vi "Read image data.vi"() -> ()   [LabVIEW 2020, in "sqlite3.lvlib"]
uses:
  sqlite3.lvlib
  sqlite/VIs/open v2.vi
  sqlite/VIs/prepare v2.vi
  sqlite/VIs/step.vi
  sqlite/VIs/column count.vi
  compound/Column.vi
  compound/Resolve Result Type.vi
  sqlite/VIs/finalize.vi
  sqlite/VIs/close v2.vi
  sqlite/subvi/Error Converter (ErrCode or Status).vi
  sqlite/VIs/column text.vi
  sqlite/VIs/column bytes.vi
  sqlite/VIs/column blob.vi
  utilities/MoveBlock.vi
  sqlite/VIs/column type.vi
  sqlite/VIs/errstr.vi
panel:
  in  "id value":string
  in  "id col":string="image"
  in  "blob column name":string="image"
  in  "table name":string="blob"
  in  "error in (no error)":errorcluster
  out "error out":errorcluster={"status"=TRUE, "code"=43, "source"="Write PNG File.vi"}
  in  "database in":path=path "C:/labview/sqlite_dbManager/test database/blob.db"
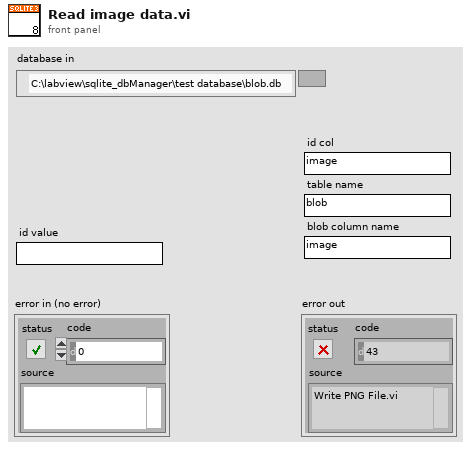
[diagram p1: front panel]
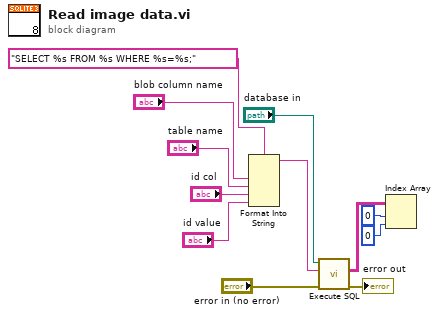
[diagram p0: block diagram]
diagram:
  n1 = Format Into String(format string="SELECT %s FROM %s WHERE %s=%s;", "blob column name", "table name", "id col", "id value") -> (resulting string=w7:string)  [unwired: 2 in, 1 out]
  n2 = call "Execute SQL.vi"("error in (no error)"="error in (no error)", "sql (string)"=w7, "database in"="database in") -> ("error out"=→"error out":errorcluster, "Query Result"=w4:string[][])  [unwired: 7 in]
  n3 = Index Array(array=w4, index (row)=0, index (col)=0 ("disabled index (col)")) -> ()  [unwired: 1 out]
